vi "Ejer 3.vi"() -> ()   [LabVIEW 2020]
panel:
  out "Numeric":dbl
  out "x*y 3":dbl
  in  "B":dbl=1000.0
  in  "A":dbl=1000.0
  out "x*y 2":ext
  out "x*y":ext
  in  "number of samples":i32=100
  in  "Stop":bool
  out "Waveform Chart":dynamicdata(graph)
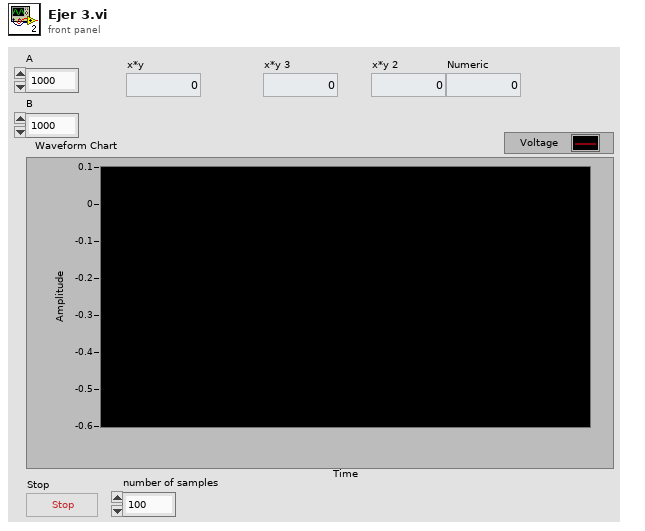
[diagram p1: front panel]
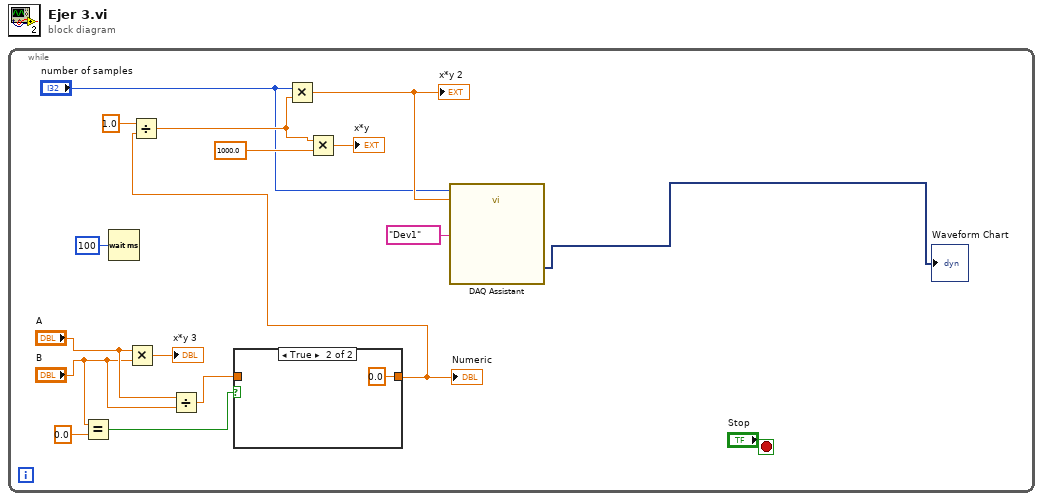
[diagram p0: block diagram]
diagram:
  n1 = while {
    stop <- "Stop" stop-if-true
    n2 = Equal?(x="B", y=0.0) -> (x = y?=w5:bool)
    n3 = Wait (ms)(milliseconds to wait=u32 100) -> ()  [unwired: 1 out]
    n4 = Multiply(x="A", y="B") -> (x*y=→"x*y 3":dbl)
    n5 = Divide(x="A", y="B") -> (x/y=w4:dbl)
    n6 = case shown="True" w5 {
      tunnel: w4 -> [w18 _]
      tunnel: [w18 0.0] -> w3
      frame False {
      }
      frame True {
      }
    }
    "Numeric" <- w3
    n7 = Divide(x=1.0, y=w3) -> (x/y=w13:dbl)
    n8 = Multiply(x="number of samples", y=w13) -> (x*y=w11:dbl)
    "x*y 2" <- w11
    n9 = Multiply(x=w13, y=1000.0) -> (x*y=→"x*y":dbl)
    n10 = call "DAQ Assistant"("rate"="number of samples", "number of samples"=w11, "device name"=tag "Dev1") -> ("data"=→"Waveform Chart":dynamicdata)  [unwired: 13 in, 3 out]
  }
